vi "禹山探头校准.vi"(5 "校准方式":u16, 6 "MB_Master输入":refnum<class "MB_Master.lvclass">, 7 "探头":T1(ring), 8 "错误输入（无错误）":errorcluster, 9 "标液三":cluster{"标准值":dbl, "检测值":dbl, "原始值":dbl}, 10 "标液二":cluster{"标准值":dbl, "检测值":dbl, "原始值":dbl}, 11 "标液一":cluster{"标准值":dbl, "检测值":dbl, "原始值":dbl}) -> (0 "错误输出":errorcluster)   [LabVIEW 2016, in "斯坦道多参数.lvlib"]
uses:
  <vilib>/Plasmionique/MB Master/MB_Master/MB_Master.lvclass
  <vilib>/Analysis/NI_AALPro.lvlib
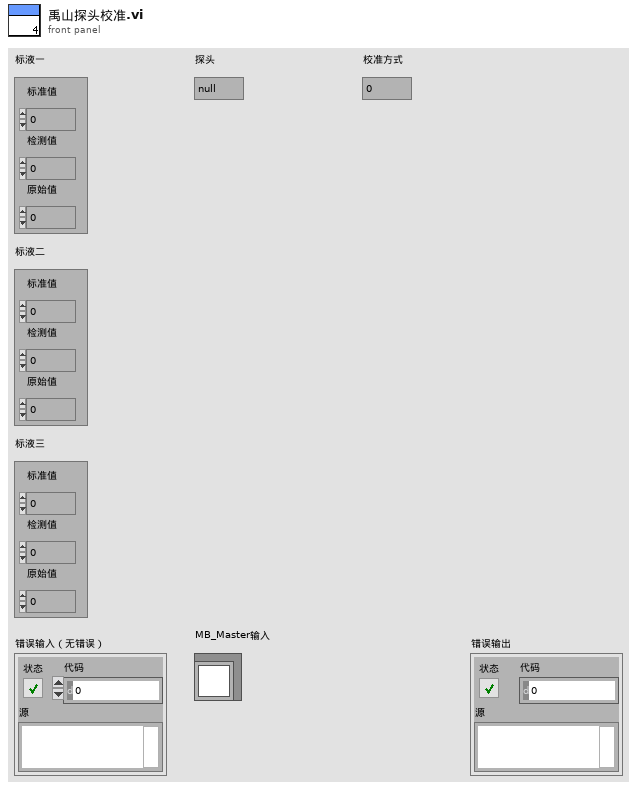
[diagram p1: front panel]
types:
  T1 = enum16{"null", "pH", "DO", "浊度", "电导率", "叶绿素a", "DO2", "藻密度"}
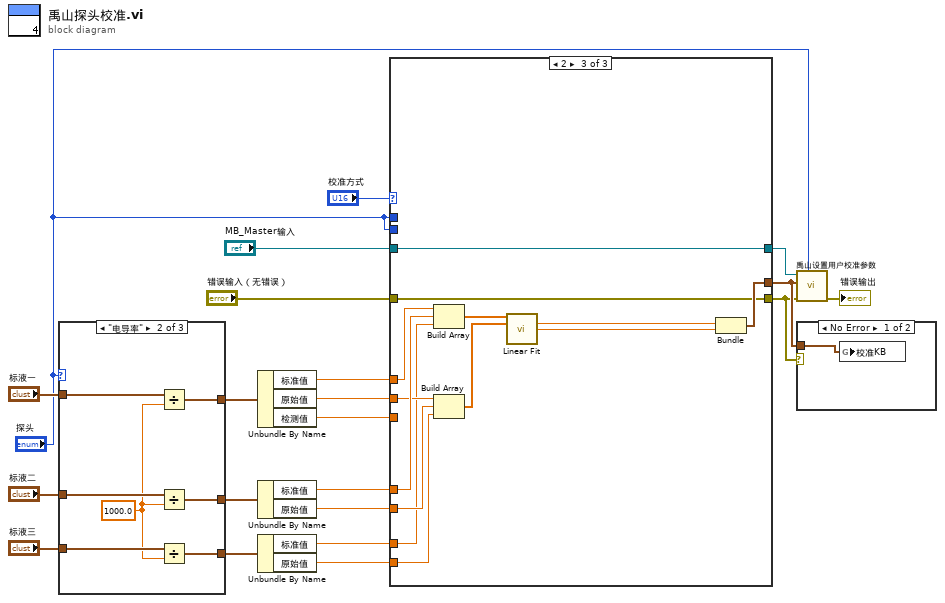
[diagram p0: block diagram]
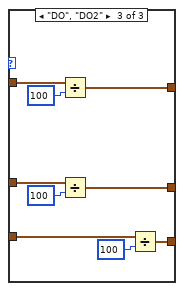
[diagram p4: hidden frame]
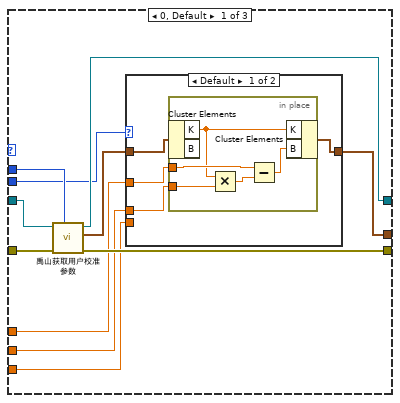
[diagram p5: hidden frame]
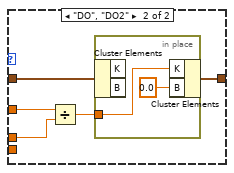
[diagram p6: hidden frame]
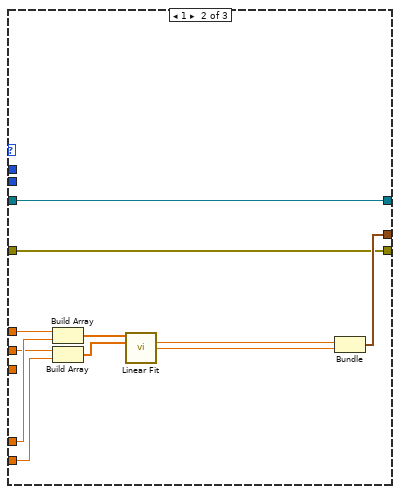
[diagram p7: hidden frame]
diagram:
  n1 = case shown="\"电导率\"" "探头" {
    tunnel: "标液三" -> [w22 w27 w40]
    tunnel: "标液二" -> [w23 w29 w39]
    tunnel: "标液一" -> [w24 w31 w38]
    tunnel: [w24 w30 w37] -> w7
    tunnel: [w23 w28 w35] -> w6
    tunnel: [w22 w26 w33] -> w5
    frame "null", Default {
    }
    frame "电导率" {
      w25 = 1000.0
      n2 = Divide(x=w31, y=w25) -> (x/y=w30:cluster{"标准值":dbl, "检测值":dbl, "原始值":dbl})
      n3 = Divide(x=w29, y=w25) -> (x/y=w28:cluster{"标准值":dbl, "检测值":dbl, "原始值":dbl})
      n4 = Divide(x=w27, y=w25) -> (x/y=w26:cluster{"标准值":dbl, "检测值":dbl, "原始值":dbl})
    }
    frame "DO", "DO2" {
      n5 = Divide(x=w38, y=100) -> (x/y=w37:cluster{"标准值":dbl, "检测值":dbl, "原始值":dbl})
      n6 = Divide(x=w39, y=100) -> (x/y=w35:cluster{"标准值":dbl, "检测值":dbl, "原始值":dbl})
      n7 = Divide(x=w40, y=100) -> (x/y=w33:cluster{"标准值":dbl, "检测值":dbl, "原始值":dbl})
    }
  }
  n8 = Unbundle By Name(w7) -> ("标准值"=w15:dbl, "原始值"=w16:dbl, "检测值"=w4:dbl)
  n9 = Unbundle By Name(w6) -> ("标准值"=w18:dbl, "原始值"=w19:dbl)
  n10 = Unbundle By Name(w5) -> ("标准值"=w20:dbl, "原始值"=w21:dbl)
  n11 = case shown="2" "校准方式" {
    tunnel: "MB_Master输入" -> [w51 w69 w82]
    tunnel: [w50 w69 w82] -> w9
    tunnel: [w49 w68 w81] -> w1
    tunnel: [w47 w70 w83] -> w2
    tunnel: "错误输入（无错误）" -> [w46 w68 w81]
    tunnel: w15 -> [w45 w78 w91]
    tunnel: w16 -> [w41 w76 w89]
    tunnel: w18 -> [_ w77 w90]
    tunnel: w19 -> [_ w75 w88]
    tunnel: w20 -> [_ _ w80]
    tunnel: w21 -> [_ _ w79]
    tunnel: "探头" -> [w44 _ _]
    tunnel: w4 -> [w43 _ _]
    tunnel: "探头" -> [w42 _ _]
    frame 0, Default {
      n12 = call "禹山获取用户校准参数.vi"("探头"=w44, "error in (no error)"=w46, "MB session in"=w51) -> ("error out"=w49:errorcluster, "输出值"=w48:cluster{"K":sgl, "B":sgl}, "MB session out"=w50:refnum<class "MB_Master.lvclass">)  [unwired: 6 in]
      n13 = case shown="Default" w42 {
        tunnel: w48 -> [w55 w65]
        tunnel: [w54 w64] -> w47
        tunnel: w45 -> [w53 w62]
        tunnel: w43 -> [_ _]
        tunnel: w41 -> [w52 w61]
        frame Default {
          n14 = in-place {
            in-place-border: w53 -> [w60]
            in-place-border: w52 -> [w59]
            n15 = in-place-cluster #1(w55) -> ("K"=w56:sgl)  [unwired: 1 out]
            n16 = Multiply(x=w56, y=w59) -> (x*y=w58:dbl)
            n17 = Subtract(x=w60, y=w58) -> (x-y=w57:dbl)
            n18 = in-place-cluster #1("K"=w56, "B"=w57) -> (w54:cluster{"K":sgl, "B":sgl})
          }
        }
        frame "DO", "DO2" {
          n19 = Divide(x=w62, y=w61) -> (x/y=w63:dbl)
          n20 = in-place {
            in-place-border: w63 -> [w67]
            n21 = in-place-cluster #2(w65) -> ()  [unwired: 2 out]
            n22 = in-place-cluster #2("K"=w67, "B"=sgl 0.0) -> (w64:cluster{"K":sgl, "B":sgl})
          }
        }
      }
    }
    frame 1 {
      n23 = Build Array(w78, w77) -> (w74:dbl[])
      n24 = Build Array(w76, w75) -> (w73:dbl[])
      n25 = call <vilib>:"Linear Fit.vi"("Y"=w74, "X"=w73) -> ("slope"=w72:dbl, "intercept"=w71:dbl)  [unwired: 9 in, 3 out]
      n26 = Bundle("slope"=w72, "intercept"=w71) -> (w70:cluster{"slope":dbl, "intercept":dbl})  [unwired: 1 in]
    }
    frame 2 {
      n27 = Build Array(w91, w90, w80) -> (w87:dbl[])
      n28 = Build Array(w89, w88, w79) -> (w86:dbl[])
      n29 = call <vilib>:"Linear Fit.vi"("Y"=w87, "X"=w86) -> ("slope"=w85:dbl, "intercept"=w84:dbl)  [unwired: 9 in, 3 out]
      n30 = Bundle("slope"=w85, "intercept"=w84) -> (w83:cluster{"slope":dbl, "intercept":dbl})  [unwired: 1 in]
    }
  }
  n31 = call "禹山设置用户校准参数.vi"("探头"="探头", "error in (no error)"=w1, "用户校准参数"=w2, "MB session in"=w9) -> ("error out"=→"错误输出":errorcluster)  [unwired: 6 in, 1 out]
  n32 = case shown="No Error" w1 {
    tunnel: w2 -> [w92 _]
    frame No Error {
      n33 = global write "多参数全局变量.vi" "校准KB"(w92) -> ()
    }
    frame Error {
    }
  }
